vi "pl1000SetPulseWidth.vi"(8 "error in (no error)":errorcluster, 9 "cycle":u8, 10 "period":u16, 11 "pl1000 handle":i16) -> (0 "error out":errorcluster, 3 "pl1000 handle out":i16)   [LabVIEW 2010]
doc: "This function sets the pulse width of the PWM (pulse-width modulated) output. \n\nperiod: the required period of the PWM waveform in microseconds, from 100 to 1800\n\ncycle: the required duty cycle as a percentage from 0 to 100"
uses:
  pl1000.dll
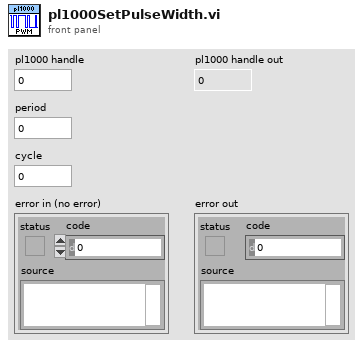
[diagram p1: front panel]
types:
  T1 = cluster{"status":bool, "code":u32, "source":string}
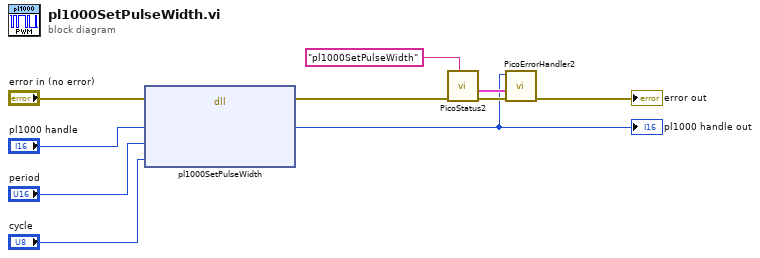
[diagram p0: block diagram]
diagram:
  n1 = dll-call lib="pl1000.dll" fn="pl1000SetPulseWidth"(error in="error in (no error)", "handle"="pl1000 handle", "period"="period", "cycle"="cycle") -> (error out=w3:errorcluster, "handle"=w1:i16)  [unwired: 5 in, 1 out]
  "pl1000 handle out" <- w1
  n2 = call "PicoStatus2.vi"("PICO source"="pl1000SetPulseWidth", "Error in"=w3) -> ("error out"=w6:errorcluster, "PICO_STATUS out"=w5:T1)  [unwired: 6 in]
  n3 = call "PicoErrorHandler2.vi"("error in (no error)"=w6, "PICO_STATUS in"=w5, "handle In"=w1) -> ("error out"=→"error out":errorcluster)  [unwired: 8 in]
